vi "Set Voltage and Current.vi"(0 "Universal Power Meter in":refnum<class "Universal Power Meter.lvclass">, 5 "Card #":u8, 7 "Voltage enum number":u16, 9 "Current enum number":u16, 11 "error in (no error)":errorcluster) -> (4 "Universal Power Meter out":refnum<class "Universal Power Meter.lvclass">, 15 "error out":errorcluster)   [LabVIEW 2013, in "Universal Power Meter.lvlib" / "Universal Power Meter.lvclass"]
uses:
  Universal Power Meter.lvclass
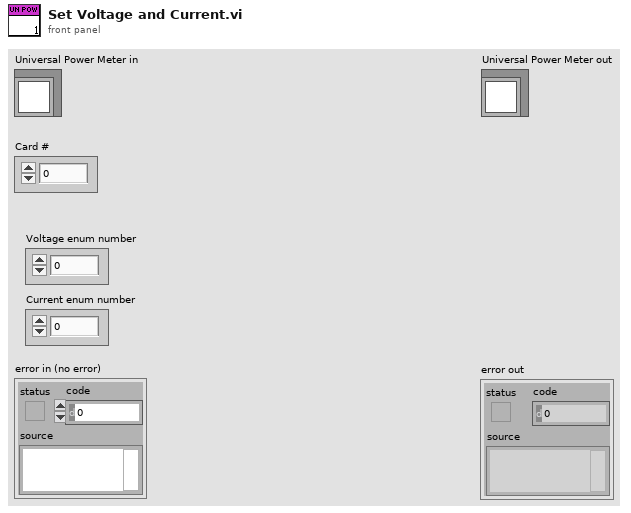
[diagram p1: front panel]
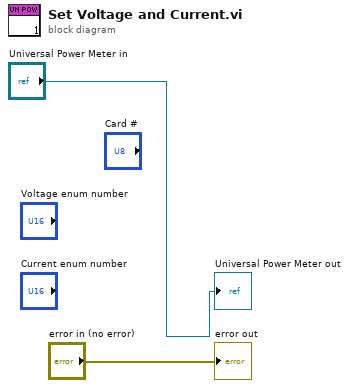
[diagram p0: block diagram]
diagram:
  "error out" <- "error in (no error)"
  "Universal Power Meter out" <- "Universal Power Meter in"
